vi "auton_picker.vi"(10 "dec_btn":bool, 11 "inc_btn":bool) -> ()   [LabVIEW 2013]
uses:
  auto_data.vi
panel:
  in  "Max Eles":u8=5
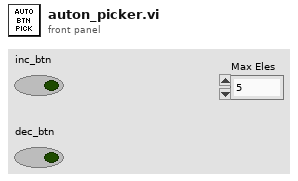
[diagram p1: front panel]
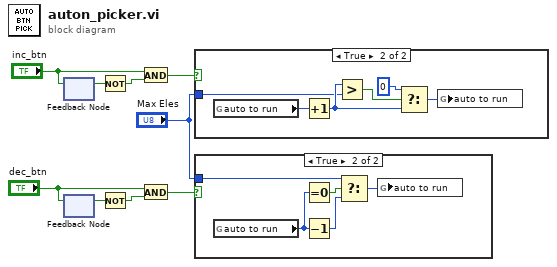
[diagram p0: block diagram]
diagram:
  n1 = feedback-in #1("inc_btn") -> ()
  n2 = feedback #1() -> (w9:bool)  [unwired: 1 in]
  n3 = feedback #2() -> (w5:bool)  [unwired: 1 in]
  n4 = feedback-in #2("dec_btn") -> ()
  n5 = Not(x=w9) -> (.not. x?=w8:bool)
  n6 = Not(x=w5) -> (.not. x?=w4:bool)
  n7 = And(x="inc_btn", y=w8) -> (x .and. y?=w6:bool)
  n8 = And(x="dec_btn", y=w4) -> (x .and. y?=w3:bool)
  n9 = case shown="True" w6 {
    tunnel: "Max Eles" -> [_ w10]
    frame False {
    }
    frame True {
      n10 = global read "auto_data.vi" "auto to run"() -> (w15:u8)
      n11 = Increment(x=w15) -> (x+1=w13:u8)
      n12 = Greater?(x=w13, y=w10) -> (0:w14:bool)
      n13 = Select(t=u8 0, s=w14, f=w13) -> (s? t:f=w11:u8)
      n14 = global write "auto_data.vi" "auto to run"(w11) -> ()
    }
  }
  n15 = case shown="True" w3 {
    tunnel: "Max Eles" -> [_ w17]
    frame False {
    }
    frame True {
      n16 = global read "auto_data.vi" "auto to run"() -> (w16:u8)
      n17 = Equal To 0?(x=w16) -> (x = 0?=w20:bool)
      n18 = Decrement(x=w16) -> (x-1=w19:u8)
      n19 = Select(t=w17, s=w20, f=w19) -> (s? t:f=w18:u8)
      n20 = global write "auto_data.vi" "auto to run"(w18) -> ()
    }
  }
